vi "AddPoint.vi"(3 "Ampitude":dbl, 5 "Freq Y":dbl, 7 "Freq X":dbl, 8 "Amp in":dbl[](array[numeric]), 9 "Y in":u32[](array[numeric]), 10 "X in":u32[](array[numeric])) -> (0 "Amp out":dbl[](array[numeric]), 1 "Y out":u32[](array[numeric]), 2 "X out":u32[](array[numeric]))   [LabVIEW 2017, in "AODControl.lvlib"]
uses:
  AODControl.lvlib
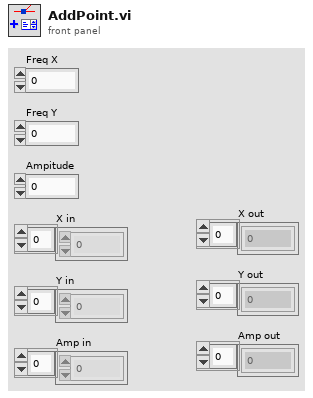
[diagram p1: front panel]
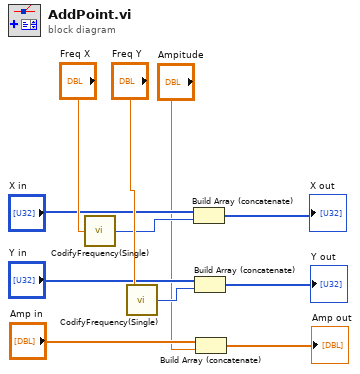
[diagram p0: block diagram]
diagram:
  n1 = call "CodifyFrequency(Single).vi"("Frequency In"="Freq X") -> ("32bit integer"=w7:u32)
  n2 = call "CodifyFrequency(Single).vi"("Frequency In"="Freq Y") -> ("32bit integer"=w4:u32)
  n3 = Build Array (concatenate)("X in", w7) -> (→"X out":u32[])
  n4 = Build Array (concatenate)("Y in", w4) -> (→"Y out":u32[])
  n5 = Build Array (concatenate)("Amp in", "Ampitude") -> (→"Amp out":dbl[])
